vi "2021_day2.vi"() -> ()   [LabVIEW 2021]
panel:
  out "Array":i32[][](array[numeric])
  out "x*y":i32
  out "array":string[](array[string])
  # "horizontal x vertical x aim"
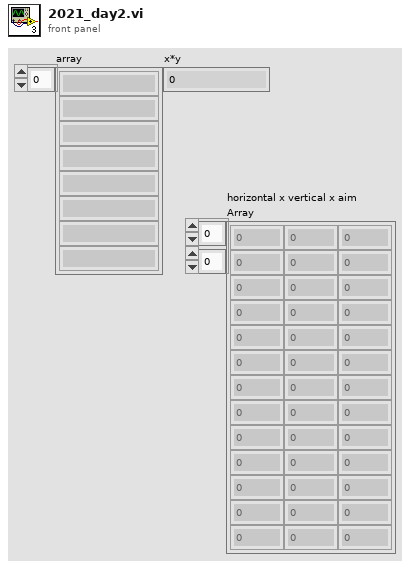
[diagram p1: front panel]
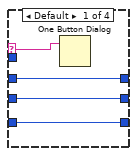
[diagram p2: hidden frame]
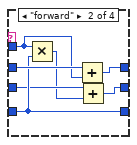
[diagram p3: hidden frame]
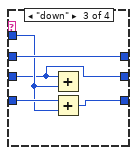
[diagram p4: hidden frame]
diagram:
  w2 = 0
  (unwired) "forward 5\ndown 5\nforward 8\nup 3\ndown 8\nforward 2"
  # "AIM"
  # "up/down"
  # "forward/backward"
  n1 = Spreadsheet String To Array(delimiter (Tab)="\n", format string="%d", spreadsheet string="forward 5\ndown 7\nforward 8\nforward 1\nforward 1\ndown 1\ndown 9\nup 4\ndown 5\ndown 3\nup 1\nup 1\nforward 1\nup 2\nforward 5\nforward 4\nforward 7\ndown 4\nup 9\nforward 5\ndown 5\nforward 2\nforward 1\nforward 3\ndown 6\nup 8\nup 8\nforward 8\nup 7\ndown 3\ndown 4\nforward 2\ndown 9\nforward 9\ndown 7\ndown 9\nforward 8\ndown 5\nforward 9\nforward 2\nforward 7\ndown 4\nforward 8\ndown 4\nup 7\nforward 7\nforward 7\nforward 5\nforward 1\ndown 1\ndown 5\nforward 9\nforward 9\ndown 2\ndown 2\ndown 2\nforward 4\nforward 3\nforward 2\ndown 7\ndown 7\nforward 8\nforward 3\nforward 1\nup 4\nforward 9\ndown 1\nup 2\nforward 3\nforward 7\nup 6\nup 9\nforward 4\ndown 8\ndown 5\ndown 9\nforward 9\nforward 4\nforward 5\nforward 3\ndown 9\nforward 1\nforward 7\ndown 5\nforward 5\nforward 3\ndown 6\ndown 5\ndown 8\nforward 6\ndown 2\nforward 2\ndown 6\nforward 1\nup 5\nup 3\nforward 7\ndown 2\nforward 2\nforward 1\nforward 9\nup 9\nup 3\nforward 5\ndown 5\nforward 9\nup 9\ndown 7\ndown 1\nup 9\ndown 7\nup 4\nforward 1\nup 2\nup 5\ndown 2\nforward 1\ndown 3\nforward 5\ndown 4\ndown 1\ndown 2\ndown 4\ndown 5\nforward 3\nforward 2\nforward 6\nforward 8\nforward 6\ndown 4\nup 7\nforward 2\ndown 3\ndown 7\ndown 1\nforward 7\nforward 1\nforward 9\nforward 8\nforward 3\nup 8\nforward 4\nup 7\nup 8\nforward 2\nforward 5\ndown 2\ndown 1\nforward 1\nup 6\ndown 7\nforward 2\nup 6\nup 2\nforward 5\ndown 5\nforward 5\nforward 3\nup 7\nforward 1\ndown 3\nforward 4\nup 5\nforward 6\nforward 1\nup 6\nup 7\nforward 1\nforward 2\nup 6\nup 6\nforward 1\nforward 5\nup 9\ndown 4\ndown 9\ndown 2\ndown 5\ndown 7\ndown 3\ndown 2\ndown 7\nforward 8\ndown 1\nforward 6\nforward 4\nup 8\nup 6\nforward 5\nforward 3\nforward 3\ndown 9\nup 1\nup 3\nup 1\nup 8\nup 9\ndown 5\ndown 5\nforward 2\nforward 5\ndown 9\ndown 1\ndown 4\nforward 5\nup 9\nforward 2\nforward 8\nup 1\ndown 9\ndown 9\ndown 2\ndown 9\nup 5\nforward 7\ndown 3\nforward 3\ndown 2\nforward 4\nforward 9\nforward 6\ndown 1\ndown 4\ndown 4\ndown 7\ndown 6\ndown 7\nforward 8\nforward 1\nforward 6\nforward 8\nup 1\ndown 2\ndown 8\nforward 4\nforward 2\ndown 1\ndown 1\ndown 9\nforward 4\ndown 3\ndown 5\ndown 7\ndown 8\nforward 9\nforward 9\nforward 4\ndown 9\ndown 5\nup 3\nup 2\nforward 9\ndown 6\nforward 4\ndown 9\nforward 9\nup 6\nup 3\nforward 3\ndown 1\nup 1\nforward 1\nforward 8\nup 4\nup 9\nforward 9\ndown 9\nup 4\ndown 4\nup 7\nforward 1\ndown 7\nforward 9\ndown 3\nforward 5\nforward 4\ndown 1\ndown 6\ndown 5\ndown 2\nforward 7\ndown 2\nforward 1\ndown 6\nforward 8\ndown 3\ndown 7\ndown 1\ndown 8\nup 4\nforward 7\nforward 9\nforward 1\nforward 9\nforward 8\nforward 9\ndown 4\nup 6\ndown 2\nup 8\ndown 7\ndown 5\nup 2\nup 7\ndown 9\nup 1\nforward 1\ndown 9\nforward 9\nforward 2\nforward 1\nup 9\ndown 5\ndown 1\nforward 7\ndown 5\nforward 6\ndown 3\nforward 2\nup 4\ndown 8\ndown 9\ndown 9\nforward 6\nforward 6\ndown 2\nforward 7\nup 2\nforward 4\ndown 6\ndown 4\nup 1\nup 5\nup 2\ndown 7\ndown 4\ndown 4\nup 7\nforward 8\nup 5\ndown 3\nforward 9\nforward 8\ndown 5\nforward 2\nup 5\ndown 6\ndown 8\nforward 2\nforward 7\nup 8\nforward 3\nup 4\nup 8\nforward 8\nforward 2\nforward 8\ndown 4\ndown 9\ndown 1\ndown 4\ndown 3\nforward 9\nforward 5\ndown 8\nforward 7\ndown 4\nup 1\ndown 4\ndown 9\nforward 4\nforward 9\ndown 8\ndown 4\ndown 2\nforward 5\nforward 2\nforward 4\nforward 4\nforward 5\ndown 4\nup 4\nup 9\ndown 7\nforward 2\nup 5\nforward 3\ndown 5\ndown 8\ndown 8\ndown 4\nforward 9\nforward 4\nforward 3\ndown 4\ndown 4\ndown 3\nup 6\nup 2\nforward 4\nup 8\ndown 1\nforward 2\nforward 4\ndown 7\nforward 7\nforward 3\ndown 3\ndown 1\nup 6\nup 7\ndown 9\nup 7\nforward 9\nforward 6\nforward 4\ndown 2\nforward 4\nforward 4\nforward 9\ndown 5\nforward 4\ndown 9\nup 9\nup 6\nforward 6\ndown 6\nforward 4\ndown 3\nforward 4\ndown 9\nup 1\ndown 5\ndown 4\nforward 4\ndown 7\ndown 3\ndown 6\ndown 5\nforward 4\nforward 3\ndown 5\nforward 6\ndown 3\nup 2\ndown 2\nup 5\ndown 4\nforward 9\nforward 1\ndown 8\nforward 8\nup 9\ndown 3\ndown 4\nforward 1\nforward 2\nup 3\ndown 9\nup 9\nforward 3\ndown 8\nforward 7\nforward 4\nforward 2\nup 9\nforward 5\nforward 7\nforward 9\nup 4\nforward 2\nforward 7\ndown 6\ndown 2\nup 5\nforward 3\ndown 8\nup 9\nforward 1\nforward 9\ndown 1\nup 3\ndown 5\nup 8\ndown 1\nforward 1\nforward 8\nforward 7\nup 9\nforward 6\nforward 5\nforward 9\ndown 2\nforward 4\ndown 9\nforward 1\nup 4\nforward 2\ndown 9\ndown 8\ndown 5\nup 9\nforward 6\ndown 7\nup 8\nforward 9\nup 5\ndown 3\nforward 2\nforward 5\nforward 6\nup 5\nforward 6\ndown 7\ndown 4\nforward 3\ndown 8\nforward 9\ndown 2\nforward 7\ndown 5\ndown 2\nforward 5\nforward 9\nforward 3\nup 3\nup 7\ndown 4\nforward 3\nup 8\nforward 8\nforward 1\ndown 4\nforward 4\nforward 2\nforward 6\nup 1\ndown 7\nforward 3\ndown 6\ndown 7\nforward 4\nforward 5\nup 9\nforward 3\nforward 6\ndown 2\ndown 1\nforward 5\nup 6\ndown 3\nforward 9\ndown 8\nup 3\nup 5\nup 6\ndown 7\nforward 1\ndown 8\nforward 7\ndown 3\nforward 1\nup 9\ndown 4\nup 9\nforward 9\ndown 4\nforward 3\nup 3\ndown 1\nup 3\nup 6\nforward 9\nforward 6\ndown 9\ndown 8\nforward 9\nup 8\ndown 8\nforward 4\nforward 3\nforward 2\ndown 6\ndown 7\ndown 1\ndown 2\ndown 2\ndown 5\nforward 8\nforward 2\ndown 4\nforward 4\ndown 5\nforward 9\nforward 1\ndown 9\nup 4\nup 5\nup 9\nforward 5\ndown 6\nup 7\nforward 1\nup 8\nup 3\nforward 2\ndown 1\nforward 3\nup 8\nup 7\ndown 8\ndown 9\nforward 7\ndown 2\nup 5\nup 8\ndown 3\nforward 3\nforward 1\nup 7\ndown 3\nup 9\ndown 8\nup 5\nforward 1\ndown 8\nup 4\nup 7\ndown 2\ndown 9\nforward 3\nup 4\nforward 4\ndown 9\nforward 1\nforward 3\nforward 9\nup 6\nforward 7\nup 8\nforward 5\ndown 2\ndown 2\nforward 4\ndown 6\nforward 7\nforward 9\nup 8\nforward 2\nup 6\nforward 6\nforward 1\nforward 5\nforward 9\nforward 5\nforward 1\nforward 8\nforward 4\nforward 1\ndown 2\nforward 3\nforward 8\nforward 6\nforward 1\ndown 7\nforward 1\nup 2\nforward 6\nup 2\nup 8\ndown 3\ndown 9\nforward 2\nforward 3\nup 9\ndown 7\nforward 6\nup 3\nforward 4\nforward 1\nup 4\ndown 1\ndown 3\ndown 7\ndown 4\nforward 4\nforward 5\nup 6\ndown 4\ndown 9\ndown 2\nforward 4\ndown 6\nforward 4\nforward 5\nforward 3\ndown 9\ndown 3\nup 8\ndown 2\ndown 8\nup 3\ndown 1\nforward 1\nforward 3\ndown 8\nup 3\nup 8\nup 1\ndown 3\ndown 9\ndown 9\ndown 6\nforward 9\ndown 7\ndown 7\ndown 4\nforward 3\nforward 3\ndown 2\ndown 6\nup 9\nforward 9\ndown 9\nforward 9\ndown 8\ndown 1\nup 3\nforward 4\nup 2\nforward 8\nup 9\nforward 8\nup 5\nforward 9\ndown 7\nforward 9\nforward 7\ndown 9\ndown 6\ndown 5\nforward 5\nforward 1\nforward 8\nup 1\nup 7\nup 5\nforward 3\ndown 1\nforward 4\nup 6\nup 3\ndown 1\nforward 4\ndown 4\nforward 4\nforward 5\ndown 2\ndown 7\ndown 1\nforward 5\nforward 2\nforward 5\nforward 1\nforward 1\ndown 7\nup 7\nforward 8\ndown 7\nforward 6\nforward 2\ndown 9\nforward 2\ndown 7\ndown 5\nup 1\ndown 6\ndown 7\ndown 6\ndown 1\nforward 5\ndown 5\nforward 6\nup 9\nforward 9\nup 1\ndown 9\nforward 4\ndown 6\ndown 2\nforward 3\ndown 9\nup 6\nforward 1\ndown 2\nforward 8\nforward 7\nforward 4\nforward 2\nforward 7\nforward 1\ndown 9\nforward 7\ndown 4\nup 6\ndown 7\nforward 1\nup 8\nforward 5\nup 3\nup 1\ndown 6\nforward 9\nup 7\nup 5\ndown 2\nup 9\nup 4\nforward 1\nforward 1\nforward 9\ndown 3\ndown 6\nforward 1\nup 6\nup 9\ndown 9\nforward 7\nforward 8\nup 9\nup 4\ndown 8\nup 3\ndown 8\nforward 9\ndown 3\ndown 6\nforward 7\nup 4\nforward 7\ndown 2\ndown 6\nup 4\ndown 8\ndown 4\ndown 2\nup 5\ndown 4\ndown 2\nforward 9\nup 9\nforward 3\ndown 9\nup 1\ndown 8\ndown 5\nforward 5\nforward 3\nup 3\nforward 9\ndown 1\nforward 1\nup 2\ndown 9\nforward 5\nforward 6\nup 3\nforward 2\nforward 8\ndown 9\nup 7\ndown 8\nup 5\nforward 9\nforward 3\ndown 7\nforward 9\ndown 8\nforward 7\ndown 6\ndown 6\ndown 1\nup 4\nup 1\nforward 3\ndown 7\nup 3\ndown 3\nforward 5\ndown 8\nforward 2\ndown 9\nforward 6\ndown 6\ndown 6\nforward 9\ndown 2\nforward 6\nup 7\ndown 3\nup 5\nforward 4\ndown 7\nforward 8\nforward 9\nforward 7\ndown 3\nforward 7\nforward 2\ndown 6\nforward 6\ndown 2\ndown 1\nforward 4\nforward 5\nup 6\nforward 7\nup 3\nup 5\nforward 2\nforward 8\nforward 9\ndown 2\nforward 4\nforward 5\ndown 7\nup 8\nforward 9\nforward 9\ndown 3\ndown 1\nforward 2\nforward 2\ndown 9\nup 5\ndown 5\nup 5\ndown 2\nforward 1\ndown 2\ndown 9\ndown 1\nforward 2\ndown 9\ndown 1\nforward 7\ndown 8\ndown 5\ndown 1\nup 5\nforward 4\ndown 8\ndown 6\ndown 6\nforward 9\nup 7\nup 2\nup 8\ndown 1\nforward 9\ndown 9\ndown 5\nforward 2\ndown 7\nup 8\nforward 5\nup 2\ndown 1\ndown 8\nup 5\nforward 1\nforward 1\ndown 7\nup 2\ndown 3\nup 6\ndown 6\nforward 7\ndown 3\nforward 8\ndown 1\ndown 4\ndown 3\nup 8\ndown 9\nup 2\nup 5\nforward 2\nforward 5\nforward 8\nup 7\nforward 4\nforward 2\nforward 2\nforward 3\nup 4\ndown 3\nforward 7\nforward 9\nforward 7", array type (2D Dbl)=string[] []) -> (array=w7:string[])
  "array" <- w7
  n2 = for {
    tunnel: w7 -> [w21] mode=indexing
    shift-right: [w14] -> w5
    shift-left: w2 -> [w17]
    shift-right: [w15] -> w6
    shift-left: w2 -> [w18]
    tunnel: [w13] -> w3 mode=indexing
    shift-right: [w11] -> _
    shift-left: w2 -> [w12]
    n3 = Scan From String(format string="%s%d", input string=w21) -> (output 1=w19:string, output 2=w16:i32)  [unwired: 4 in, 3 out]
    n4 = case shown="\"up\"" w19 {
      selector: w19 -> [w23 _ _ _]
      tunnel: [w25 w31 w37 w42] -> w15
      tunnel: w18 -> [w25 w32 w37 w42]
      tunnel: [w24 w28 w33 w38] -> w14
      tunnel: w17 -> [w24 w29 w33 w38]
      tunnel: w16 -> [_ w26 w34 w39]
      tunnel: [w22 w30 w35 w40] -> w11
      tunnel: w12 -> [w22 w30 w36 w41]
      frame Default {
        n5 = One Button Dialog(message=w23) -> ()  [unwired: 1 in, 1 out]
      }
      frame "forward" {
        n6 = Multiply(x=w26, y=w30) -> (x*y=w27:i32)
        n7 = Add(x=w32, y=w26) -> (x+y=w31:i32)
        n8 = Add(x=w29, y=w27) -> (x+y=w28:i32)
      }
      frame "down" {
        n9 = Add(x=w33, y=w34) -> ()  [unwired: 1 out]
        n10 = Add(x=w36, y=w34) -> (x+y=w35:i32)
      }
      frame "up" {
        n11 = Subtract(x=w38, y=w39) -> ()  [unwired: 1 out]
        n12 = Subtract(x=w41, y=w39) -> (x-y=w40:i32)
      }
    }
    n13 = Build Array(w15, w14, w11) -> (w13:i32[])
  }
  "Array" <- w3
  n14 = Multiply(x=w6, y=w5) -> (x*y=→"x*y":i32)
